vi "mirrorswitch_move.vi"(2 "RetPos":bool, 3 "Wait":bool=TRUE, 4 "GoTo (mm)":sgl, 5 "MG17Motor":refnum<k7>(container)) -> (0 "StartPosition(um)":sgl, 1 "EndPosition (um)":sgl)   [LabVIEW 2015]
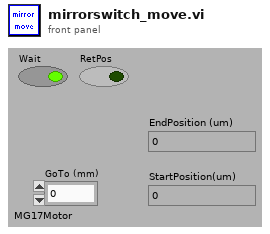
[diagram p1: front panel]
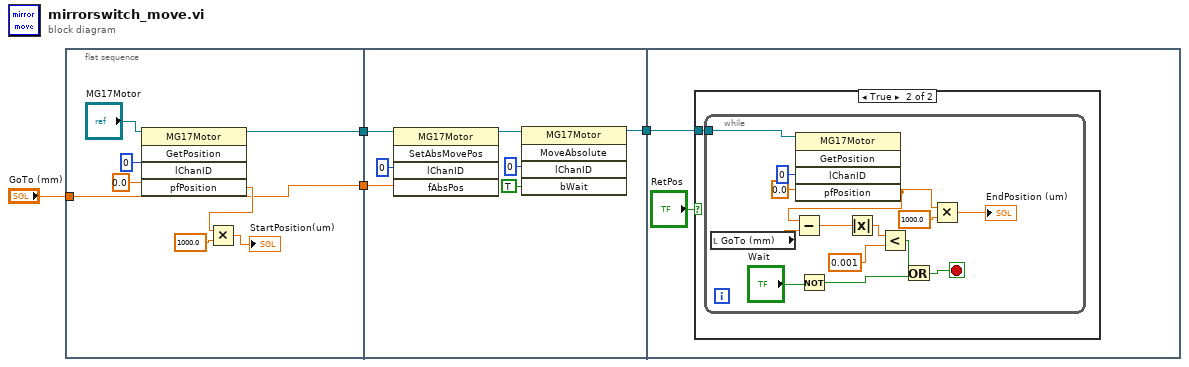
[diagram p0: block diagram]
diagram:
  n1 = flat-sequence {
    tunnel: [w11] -> w4
    tunnel: [w6] -> w3
    tunnel: "GoTo (mm)" -> [w6]
    tunnel: w4 -> [w19]
    tunnel: w3 -> [w17]
    tunnel: [w13] -> w2
    tunnel: w2 -> [w21]
    frame #0 {
      n2 = invoke class="MG17Motor" method="GetPosition"(reference="MG17Motor", "lChanID"=0, "pfPosition"=sgl 0.0) -> (reference out=w11:refnum<k7>, "pfPosition"=w9:sgl)  [unwired: 2 in, 3 out]
      n3 = Multiply(x=w9, y=sgl 1000.0) -> (x*y=→"StartPosition(um)":sgl)
    }
    frame #1 {
      n4 = invoke class="MG17Motor" method="SetAbsMovePos"(reference=w19, "lChanID"=0, "fAbsPos"=w17) -> (reference out=w18:refnum<k7>)  [unwired: 2 in, 4 out]
      n5 = invoke class="MG17Motor" method="MoveAbsolute"(reference=w18, "lChanID"=0, "bWait"=TRUE) -> (reference out=w13:refnum<k7>)  [unwired: 2 in, 4 out]
    }
    frame #2 {
      n6 = case shown="True" "RetPos" {
        tunnel: w21 -> [_ w22]
        frame False {
        }
        frame True {
          n7 = while {
            tunnel: w22 -> [w31]
            stop <- w23 stop-if-true
            n8 = local read "GoTo (mm)"() -> (w27:sgl)
            n9 = invoke class="MG17Motor" method="GetPosition"(reference=w31, "lChanID"=0, "pfPosition"=sgl 0.0) -> ("pfPosition"=w29:sgl)  [unwired: 2 in, 4 out]
            n10 = Subtract(x=w29, y=w27) -> (x-y=w34:sgl)
            n11 = Not(x="Wait") -> (.not. x?=w25:bool)
            n12 = Absolute Value(x=w34) -> (abs(x)=w33:sgl)
            n13 = Less?(x=w33, y=0.001) -> (x < y?=w24:bool)
            n14 = Or(x=w24, y=w25) -> (x .or. y?=w23:bool)
            n15 = Multiply(x=w29, y=sgl 1000.0) -> (x*y=→"EndPosition (um)":sgl)
          }
        }
      }
    }
  }
